vi "FTW-Panel-FrontPanel-SetCursor.vi"(8 "error in":errorcluster, 10 "Cursor":enum32{"Default", "Busy", "Unset Busy", "Link"}(ring), 11 "VI Ref":refnum<vi>) -> (0 "error out":errorcluster, 3 "VI Ref out":refnum<vi>)   [LabVIEW 2012]
panel:
  # "Inputs"
  # "Outputs"
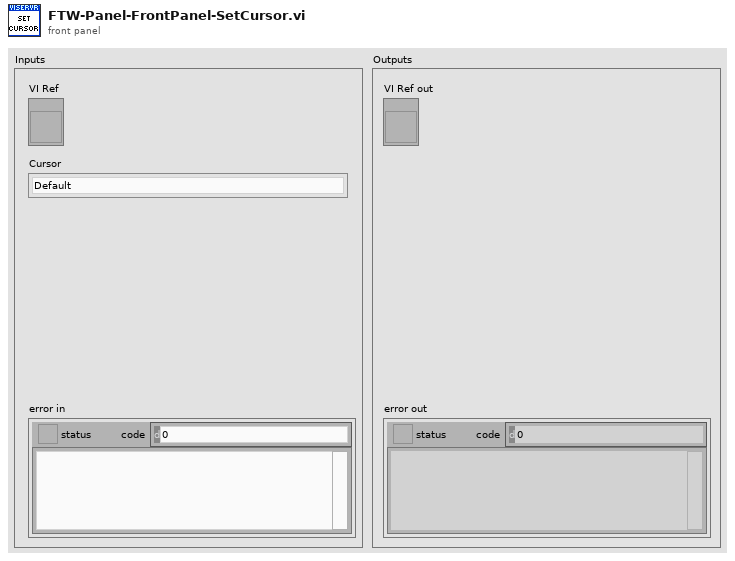
[diagram p1: front panel]
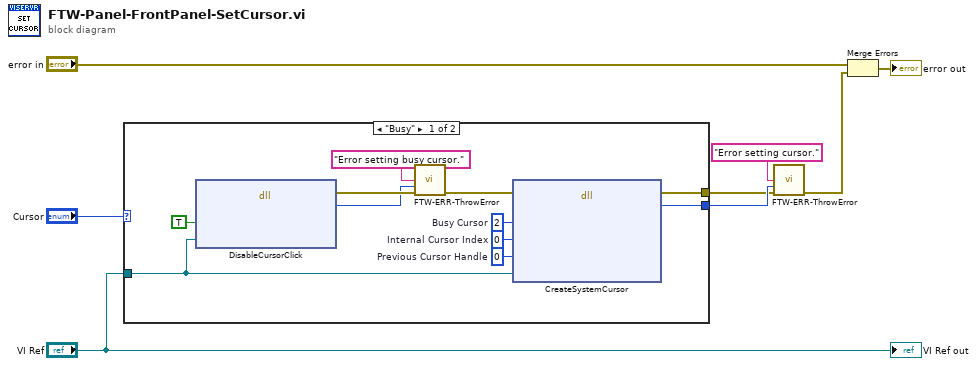
[diagram p0: block diagram]
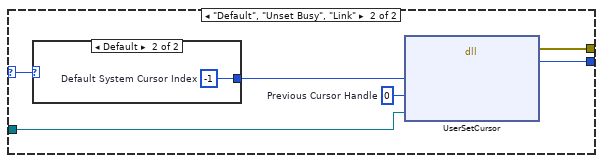
[diagram p2: hidden frame]
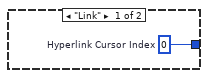
[diagram p3: hidden frame]
diagram:
  n1 = case shown="\"Busy\"" "Cursor" {
    selector: "Cursor" -> [_ w21]
    tunnel: "VI Ref" -> [w9 w25]
    tunnel: [w10 w24] -> w6
    tunnel: [w11 w23] -> w5
    frame "Busy" {
      w12 = 0  # Internal Cursor Index
      w13 = 0  # Previous Cursor Handle
      w14 = 2  # Busy Cursor
      n2 = dll-call lib="LabVIEW" fn="DisableCursorClick"("Disable Click?"=TRUE, "VI Ref"=w9) -> (error out=w18:errorcluster, "Return"=w17:i32)  [unwired: 5 in, 1 out]
      n3 = call "FTW-ERR-ThrowError.vi"("Error Message"="Error setting busy cursor.", "Error Code"=w17, "error in"=w18) -> ("error out"=w15:errorcluster)  [unwired: 12 in]
      n4 = dll-call lib="LabVIEW" fn="CreateSystemCursor"(error in=w15, "Cursor Index"=w14, "Internal Cursor Index"=w12, "Previous Cursor Handle"=w13, "VI Ref"=w9) -> (error out=w11:errorcluster, "Return"=w10:i32)  [unwired: 6 in, 1 out]
    }
    frame "Default", "Unset Busy", "Link" {
      w22 = 0  # Previous Cursor Handle
      n5 = case shown="Default" w21 {
        tunnel: [w26 w27] -> w20
        frame "Link" {
          w26 = 0  # Hyperlink Cursor Index
        }
        frame Default {
          w27 = -1  # Default System Cursor Index
        }
      }
      n6 = dll-call lib="LabVIEW" fn="UserSetCursor"("Internal Cursor Index"=w20, "Previous Cursor Handle"=w22, "VI Ref"=w25) -> (error out=w23:errorcluster, "Return"=w24:i32)  [unwired: 6 in, 1 out]
    }
  }
  n7 = call "FTW-ERR-ThrowError.vi"("Error Message"="Error setting cursor.", "Error Code"=w6, "error in"=w5) -> ("error out"=w1:errorcluster)  [unwired: 12 in]
  n8 = Merge Errors("error in", w1) -> (→"error out":errorcluster)
  "VI Ref out" <- "VI Ref"
